vi "3D Line Graph.vi"() -> ()   [LabVIEW 2020]
uses:
  <vilib>/Native 3D Graph/xcontrol/3DPC_SurfacePlot.xctl
panel:
  out "3D Graph":refnum<class "Base Datatype.lvclass">[](xcontrol)
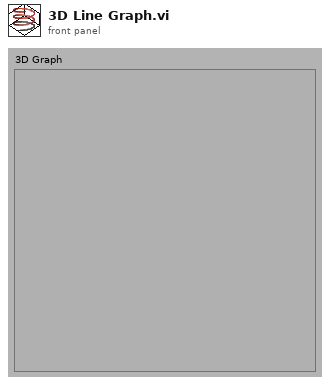
[diagram p1: front panel]
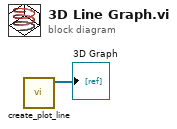
[diagram p0: block diagram]
diagram:
  n1 = call <vilib>:"create_plot_line.vi"() -> ("plots out"=→"3D Graph":refnum<class "Base Datatype.lvclass">[])  [unwired: 5 in, 6 out]
